vi "Query Sys (To) Parameters.vi"   [LabVIEW 2013, in "Berkeley Nucleonics 500 Series.lvlib"]
doc: "This polymorphic VI contains VIs to read the mode configuration of the system timer (To)."
uses:
  Berkeley Nucleonics 500 Series.lvlib
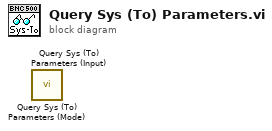
[diagram p0: block diagram]
diagram:
  n1 = call "Query Sys (To) Parameters (Mode).vi"() -> ()  [unwired: 9 in, 3 out]
  n2 = call "Query Sys (To) Parameters (Input).vi"() -> ()  [unwired: 9 in, 3 out]
